vi "svx_Timebase Graph Type Change.vi"(8 "Container Bounds In":T2, 10 "Prev Graph Type":T3, 11 "Graph Type":T3) -> (0 "Container Bounds Out":T2)   [LabVIEW 2017, in "SVX Timebase.xctl"]
uses:
  <vilib>/addons/_XControls/Timebase Plot/SVX Timebase.xctl
  <vilib>/addons/_XControls/Timebase Plot/subVIs/svx_Timebase Graph Types.ctl
  <vilib>/addons/_XControls/Timebase Plot/subVIs/svx_Timebase Bounds.ctl
panel:
  out "X axis":T1(graph)
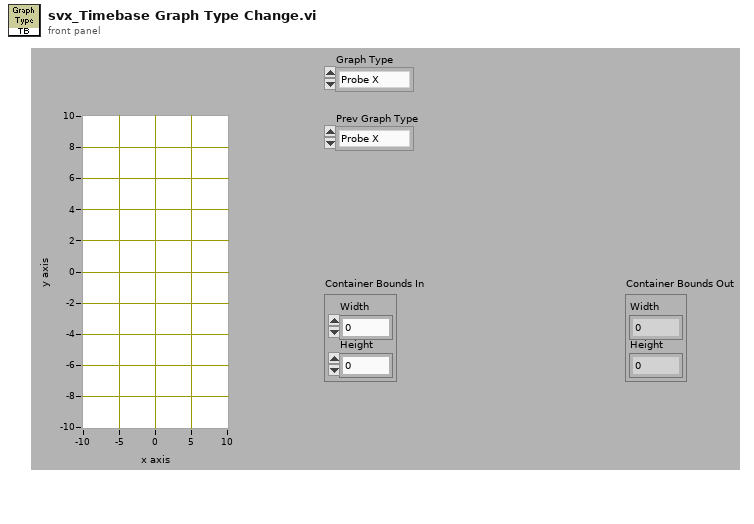
[diagram p1: front panel]
types:
  T1 = cluster{"orbit plot X":dbl[], "orbit plot Y":dbl[]}[]
  T2 = typedef "SVX Timebase.xctl/svx_Timebase Bounds.ctl" = cluster{"Width":u32, "Height":u32}
  T3 = typedef "SVX Timebase.xctl/svx_Timebase Graph Types.ctl" = enum16{"Probe X", "Probe Y", "Probe X and Y"}
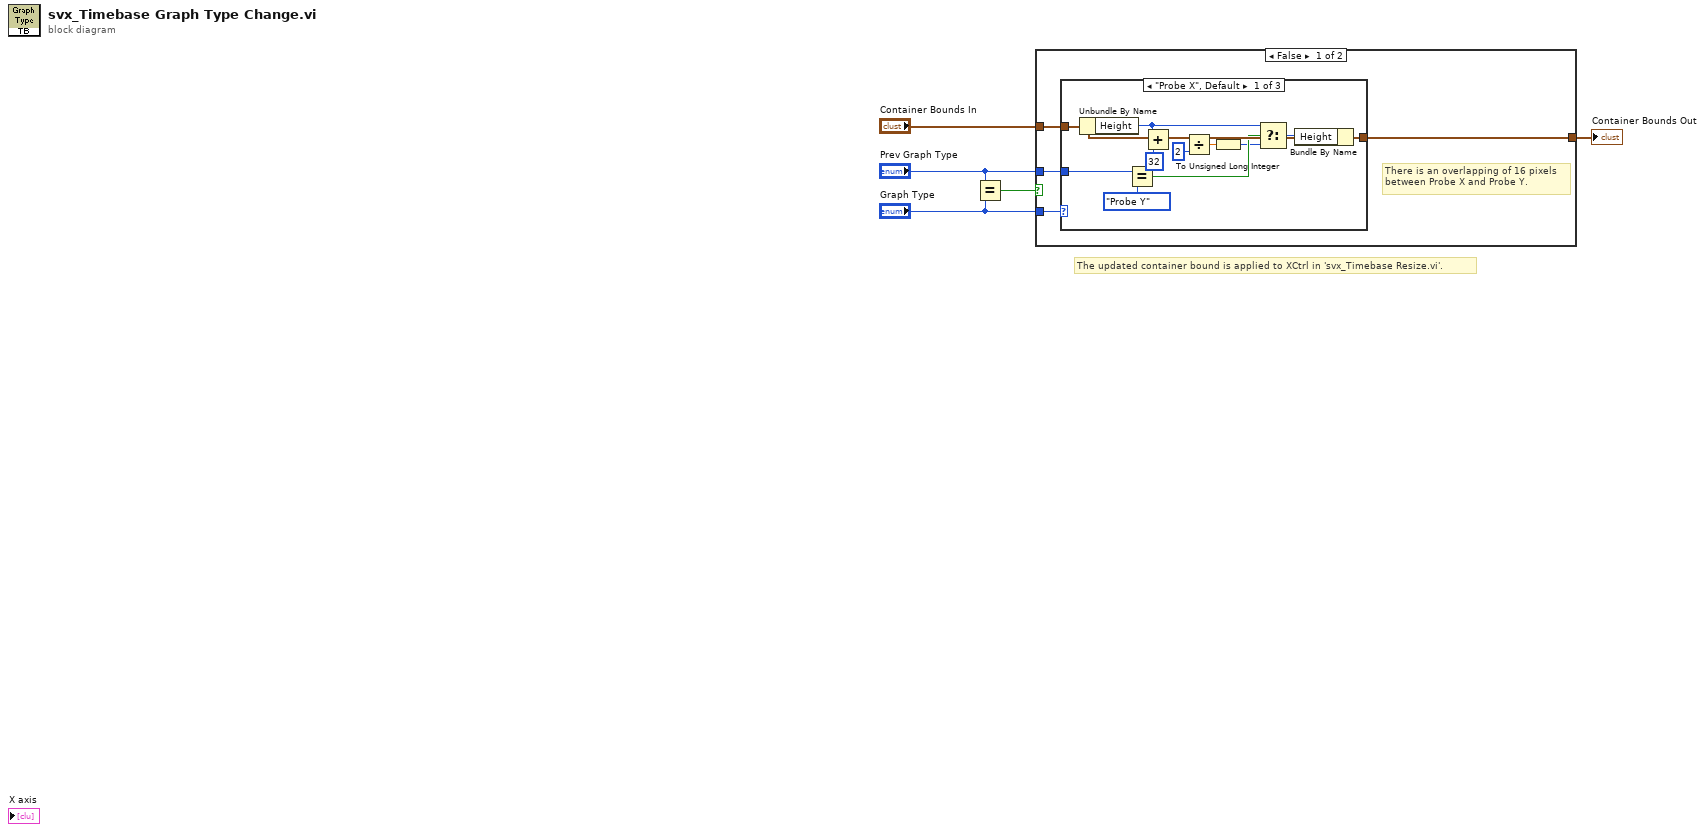
[diagram p0: block diagram]
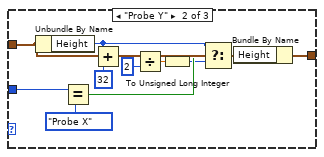
[diagram p2: hidden frame]
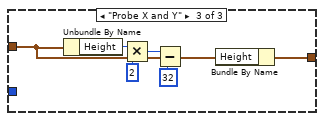
[diagram p3: hidden frame]
diagram:
  # "The updated container bound is applied to XCtrl in 'svx_Timebase Resize.vi'."
  n1 = Equal?(x="Graph Type", y="Prev Graph Type") -> (x = y?=w5:bool)
  n2 = case shown="False" w5 {
    tunnel: "Graph Type" -> [w9 _]
    tunnel: "Prev Graph Type" -> [w7 _]
    tunnel: "Container Bounds In" -> [w8 w41]
    tunnel: [w6 w41] -> w2
    frame False {
      # "There is an overlapping of 16 pixels\nbetween Probe X and Probe Y."
      n3 = case shown="\"Probe X\", Default" w9 {
        tunnel: w8 -> [w18 w30 w38]
        tunnel: [w19 w31 w37] -> w6
        tunnel: w7 -> [w14 w26 _]
        frame "Probe X", Default {
          n4 = Unbundle By Name(w18) -> ("Height"=w11:u32)
          n5 = Equal?(x=w14, y=svx_Timebase_Graph_Types."Probe Y" ("Graph Type")) -> (x = y?=w17:bool)
          n6 = Add(x=w11, y=u32 32) -> (x+y=w10:u32)
          n7 = Divide(x=w10, y=u32 2) -> (x/y=w20:dbl)
          n8 = To Unsigned Long Integer(number=w20) -> (unsigned 32bit integer=w12:u32)
          n9 = Select(t=w11, s=w17, f=w12) -> (s? t:f=w16:u32)
          n10 = Bundle By Name(cluster=w18, "Height"=w16) -> (w19:T2)
        }
        frame "Probe Y" {
          n11 = Unbundle By Name(w30) -> ("Height"=w23:u32)
          n12 = Equal?(x=w26, y=svx_Timebase_Graph_Types."Probe X" ("Graph Type")) -> (x = y?=w29:bool)
          n13 = Add(x=w23, y=u32 32) -> (x+y=w22:u32)
          n14 = Divide(x=w22, y=u32 2) -> (x/y=w32:dbl)
          n15 = To Unsigned Long Integer(number=w32) -> (unsigned 32bit integer=w24:u32)
          n16 = Select(t=w23, s=w29, f=w24) -> (s? t:f=w28:u32)
          n17 = Bundle By Name(cluster=w30, "Height"=w28) -> (w31:T2)
        }
        frame "Probe X and Y" {
          n18 = Unbundle By Name(w38) -> ("Height"=w40:u32)
          n19 = Multiply(x=w40, y=u32 2) -> (x*y=w36:u32)
          n20 = Subtract(x=w36, y=u32 32) -> (x-y=w34:u32)
          n21 = Bundle By Name(cluster=w38, "Height"=w34) -> (w37:T2)
        }
      }
    }
    frame True {
    }
  }
  "Container Bounds Out" <- w2
